vi "SetResolution.vi"(8 "error in (no error)":errorcluster, 10 "Input: Resolution - H/L":string="\r", 11 "Serial Controller in":refnum<class "Serial Controller.lvclass">) -> (0 "error out":errorcluster, 3 "Serial Controller out":refnum<class "Serial Controller.lvclass">)   [LabVIEW 2014, in "Serial Controller.lvclass"]
uses:
  Serial Controller.lvclass
  Serial Controller.lvclass/Serial Controller.ctl
panel:
  out "Read":bool
  out "Serial Read":string
  out "Output: Resolution":bool
  out "Output: Resolution - H/L":string
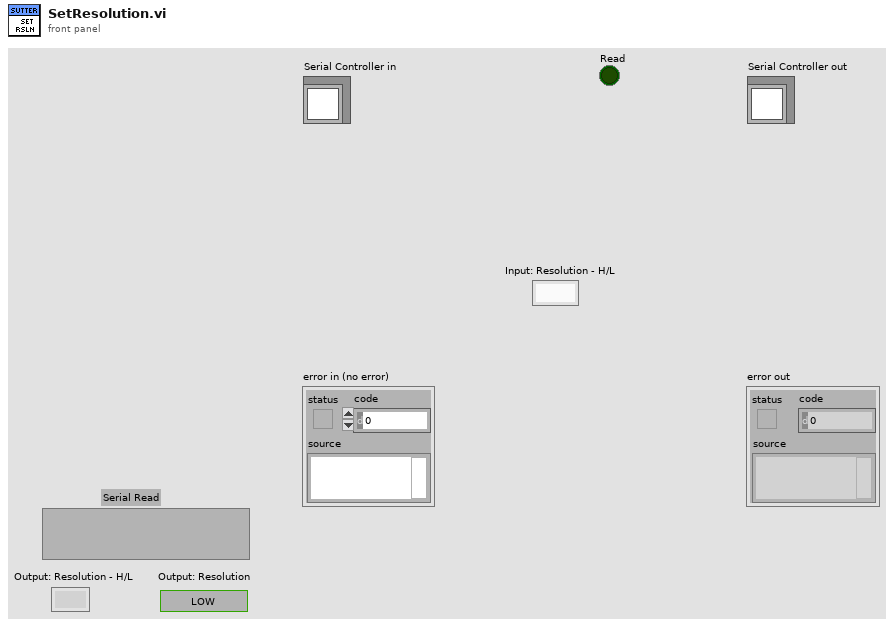
[diagram p1: front panel]
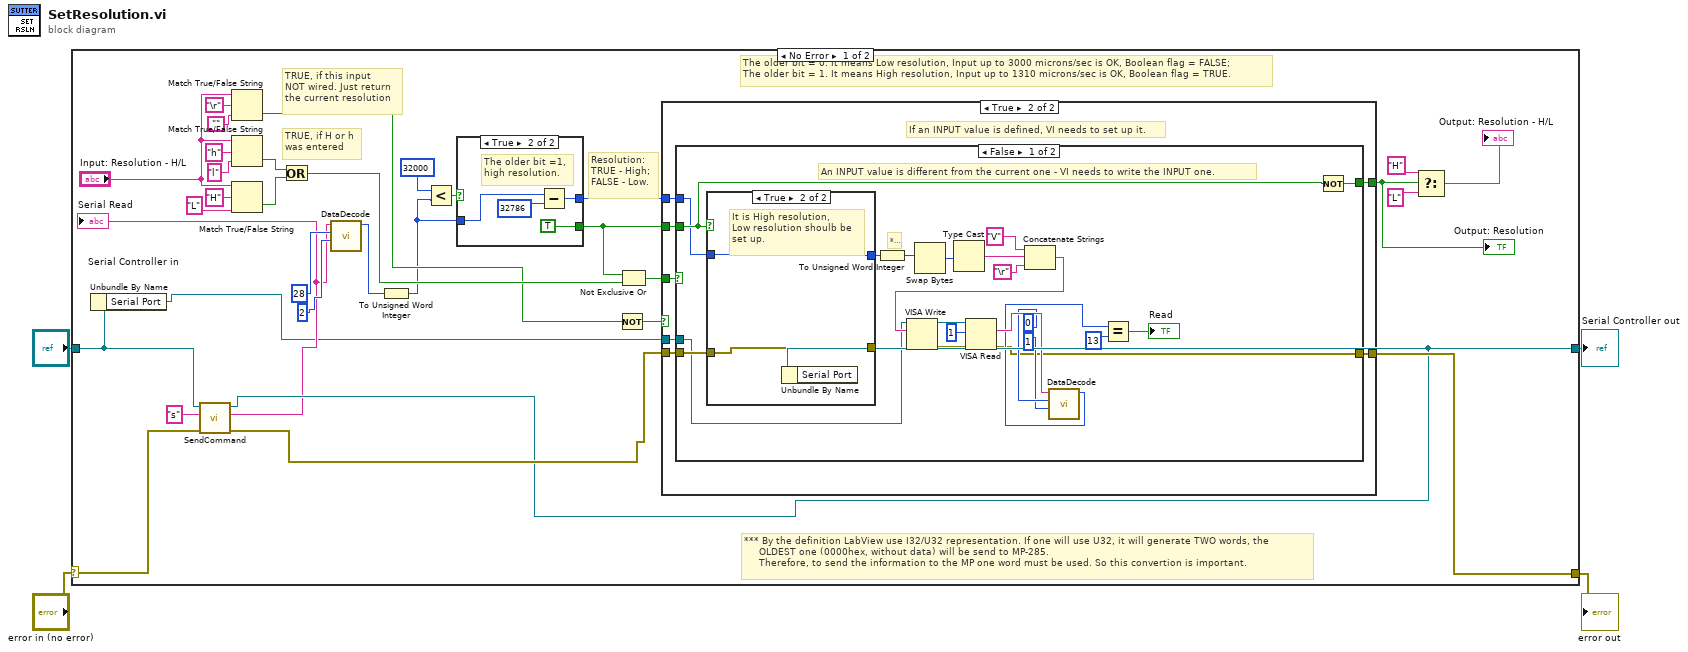
[diagram p0: block diagram]
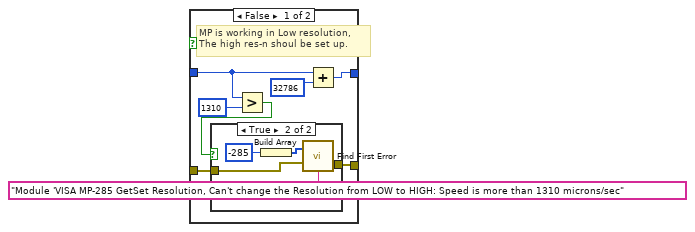
[diagram p3: hidden frame]
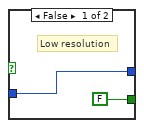
[diagram p6: hidden frame]
diagram:
  n1 = case shown="No Error" "error in (no error)" {
    selector: "error in (no error)" -> [w10 w94]
    tunnel: [w15 w94] -> w3
    tunnel: [w8 w93] -> w2
    tunnel: "Serial Controller in" -> [w6 w93]
    frame No Error {
      # "TRUE, if this input\nNOT wired. Just return\nthe current resolution"
      # "TRUE, if H or h\nwas entered"
      # "*** By the definition LabView use I32/U32 representation. If one will use U32, it will generate TWO words, the \n     OLDEST one (0000hex, without data) will be send to MP-285. \n     Therefore, to send the information to the MP one word must be used. So this convertion is important."
      # "The older bit = 0. It means Low resolution, Input up to 3000 microns/sec is OK, Boolean flag = FALSE;\nThe older bit = 1. It means High resolution, Input up to 1310 microns/sec is OK, Boolean flag = TRUE."
      # "Resolution:\nTRUE - High;\nFALSE - Low."
      n2 = Unbundle By Name(w6) -> ("Serial Port"=w5:refnum<visa-resource-name>)
      n3 = call-dynamic "SendCommand.vi"("error in (no error)"=w10, "command"="s", "Serial Controller in"=w6) -> ("error out"=w9:errorcluster, "Returned"=w7:string, "Serial Controller out"=w8:refnum<class "Serial Controller.lvclass">)  [unwired: 6 in]
      "Serial Read" <- w7
      n4 = Match True/False String(2:"", 3:"\r", 4:"Input: Resolution - H/L") -> (0:w27:bool)  [unwired: 1 out]
      n5 = Match True/False String(2:"l", 3:"h", 4:"Input: Resolution - H/L") -> (0:w22:bool)  [unwired: 1 out]
      n6 = Match True/False String(2:"L", 3:"H", 4:"Input: Resolution - H/L") -> (0:w23:bool)  [unwired: 1 out]
      n7 = Or(x=w22, y=w23) -> (x .or. y?=w29:bool)
      n8 = call "DataDecode.vi"("Input: lenght"=2 ("length"), "Input: offset"=28 ("offset (0)"), "Input: Data string"=w7) -> ("Output: Decoded Data"=w12:i32)  [unwired: 4 in]
      n9 = To Unsigned Word Integer(number=w12) -> (unsigned 16bit integer=w18:u16)
      n10 = Less?(x=32000, y=w18) -> (x < y?=w16:bool)
      n11 = case shown="True" w16 {
        tunnel: [w88 w92] -> w19
        tunnel: w18 -> [w88 w90]
        tunnel: [FALSE TRUE] -> w30
        frame False {
          # "Low resolution"
        }
        frame True {
          # "The older bit =1, \nhigh resolution."
          n12 = Subtract(x=w90, y=32786) -> (x-y=w92:i32)
        }
      }
      n13 = Not(x=w27) -> (.not. x?=w26:bool)
      n14 = Not Exclusive Or(1:w29, 2:w30) -> (0:w28:bool)
      n15 = case shown="True" w26 {
        tunnel: w5 -> [_ w46]
        tunnel: w9 -> [w39 w45]
        tunnel: [w39 w44] -> w15
        tunnel: w30 -> [w38 w43]
        tunnel: w19 -> [_ w41]
        tunnel: w28 -> [_ w42]
        tunnel: [w38 w40] -> w37
        frame False {
          # "If an INPUT value was not seted up there is nothing to write, just output the current Resolution."
        }
        frame True {
          # "If an INPUT value is defined, VI needs to set up it."
          n16 = case shown="False" w42 {
            tunnel: w45 -> [w55 w86]
            tunnel: w46 -> [w54 _]
            tunnel: [w47 w86] -> w44
            tunnel: w43 -> [w58 w85]
            tunnel: [w57 w85] -> w40
            tunnel: w41 -> [w56 _]
            frame False {
              # "***"
              # "An INPUT value is different from the current one - VI needs to write the INPUT one."
              n17 = case shown="True" w58 {
                tunnel: w56 -> [w74 w84]
                tunnel: [w76 w84] -> w60
                tunnel: w55 -> [w70 w83]
                tunnel: [w71 w83] -> w53
                frame False {
                  # "MP is working in Low resolution,\nThe high res-n shoul be set up."
                  n18 = Greater?(x=w74, y=1310) -> (0:w72:bool)
                  n19 = case shown="True" w72 {
                    tunnel: [w77 w79] -> w71
                    tunnel: w70 -> [w77 w78]
                    frame False {
                    }
                    frame True {
                      n20 = Build Array(-285) -> (w81:i32[])
                      n21 = call <vilib>:"Find First Error.vi"("error in (no error)"=w78, "source messages"="Module 'VISA MP-285 GetSet Resolution, Can't change the Resolution from LOW to HIGH: Speed is more than 1310 microns/sec", "error codes"=w81) -> ("error out"=w79:errorcluster)  [unwired: 2 out]
                    }
                  }
                  n22 = Add(x=w74, y=32786) -> (x+y=w76:i32)
                }
                frame True {
                  # "It is High resolution,\nLow resolution shoulb be\nset up."
                }
              }
              n23 = To Unsigned Word Integer(number=w60) -> (unsigned 16bit integer=w59:u16)
              n24 = Swap Bytes(anything=w59) -> (byte swapped=w62:u16)
              n25 = Type Cast(x=w62) -> (*(type *) &x=w61:string)  [unwired: 1 out]
              n26 = Concatenate Strings("V", w61, "\r") -> (w68:string)
              n27 = VISA Write(VISA resource name=w54, write buffer=w68, error in (no error)=w53) -> (VISA resource name out=w67:refnum<visa-resource-name>, error out=w66:errorcluster)  [unwired: 1 out]
              n28 = VISA Read(VISA resource name=w67, byte count=1, error in (no error)=w66) -> (read buffer=w52:string, error out=w47:errorcluster)  [unwired: 2 out]
              n29 = call "DataDecode.vi"("Input: lenght"=1, "Input: offset"=0, "Input: Data string"=w52) -> ("Output: Decoded Data"=w49:i32)  [unwired: 4 in]
              n30 = Equal?(x=w49, y=13) -> (x = y?=→"Read":bool)
              n31 = Not(x=w58) -> (.not. x?=w57:bool)
            }
            frame True {
              # "An INPUT value is the same, as current one --> Nothing to do!"
            }
          }
        }
      }
      "Output: Resolution" <- w37
      n32 = Unbundle By Name(w8) -> ()  [unwired: 1 out]
      n33 = Select(t="H", s=w37, f="L") -> (s? t:f=→"Output: Resolution - H/L":string)
    }
    frame Error {
    }
  }
  "error out" <- w3
  "Serial Controller out" <- w2
